vi "openSession.vi"(2 "error in (no error)":errorcluster, 3 "BK1823ACounter.lvclass":refnum<class "BK1823ACounter.lvclass">) -> (0 "error out":errorcluster, 1 "BK1823ACounter.lvclass 2":refnum<class "BK1823ACounter.lvclass">)   [LabVIEW 2011, in "Hardware.lvlib" / "frequencyCounters.lvlib" / "BK1823ACounter.lvclass"]
uses:
  BK1823ACounter.lvclass
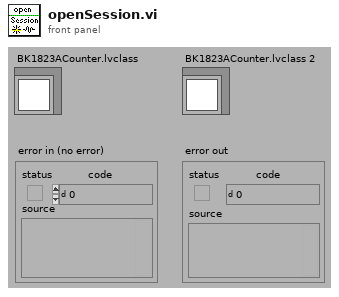
[diagram p1: front panel]
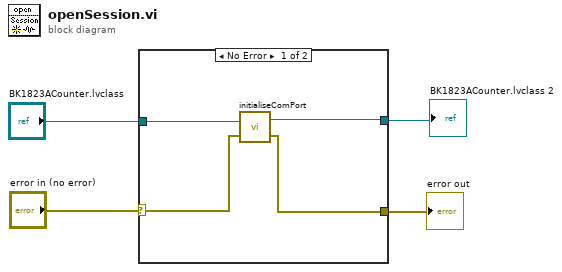
[diagram p0: block diagram]
diagram:
  n1 = case shown="No Error" "error in (no error)" {
    selector: "error in (no error)" -> [w5 w9]
    tunnel: "BK1823ACounter.lvclass" -> [w8 w10]
    tunnel: [w7 w10] -> w3
    tunnel: [w6 w9] -> w2
    frame No Error {
      n2 = call "initialiseComPort.vi"("error in (no error)"=w5, "BK1823ACounter.lvclass"=w8) -> ("error out"=w6:errorcluster, "BK1823ACounter.lvclass 2"=w7:refnum<class "BK1823ACounter.lvclass">)
    }
    frame Error {
    }
  }
  "BK1823ACounter.lvclass 2" <- w3
  "error out" <- w2
